vi "rotina_injecao_1.0.vi"() -> ()   [LabVIEW 2011]
panel:
  out "Cicles":i32
  in  "return valve (min)":dbl=1.1 caption="Time Target (s)"
  in  "#  Clicles":i32=3
  in  "stop air valve (s)":dbl=4.0 caption="Time Target (s)"
  in  "Time to get ready":dbl=0.5 caption="Time Target (s)"
  in  "Chromatogram Time (min)":dbl=2.0 caption="Time Target (s)"
  in  "Boolean":bool=TRUE
  out "TCD":dbl(graph)
  out "Time has Elapsed":bool
  out "Elapsed Time (min)":dbl caption="Elapsed Time (s)"
  out "Counter":i32
  out "FID":cluster{"value":dbl}(graph)
  out "date string":string
  out "time string":string
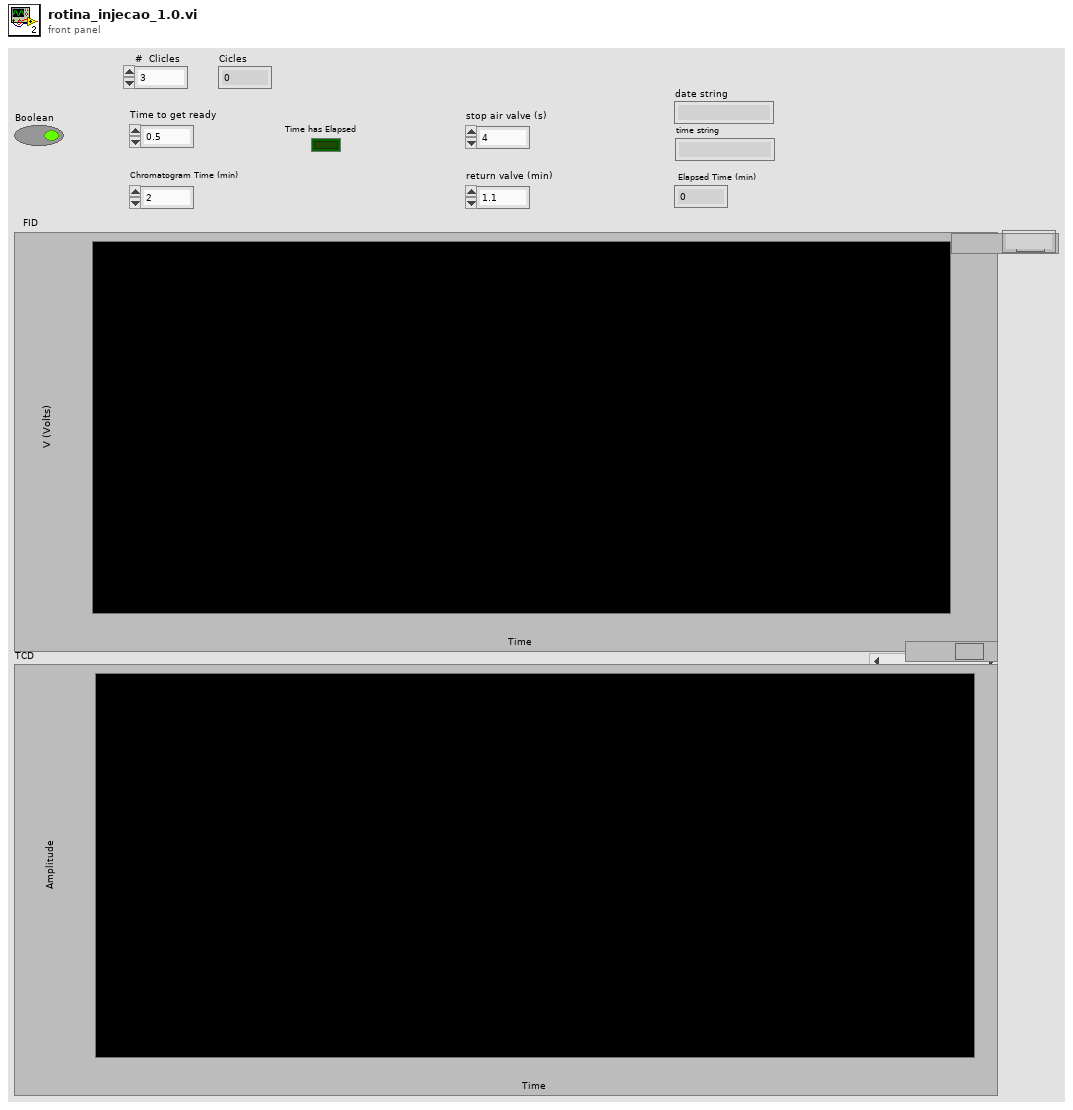
[diagram p1: front panel]
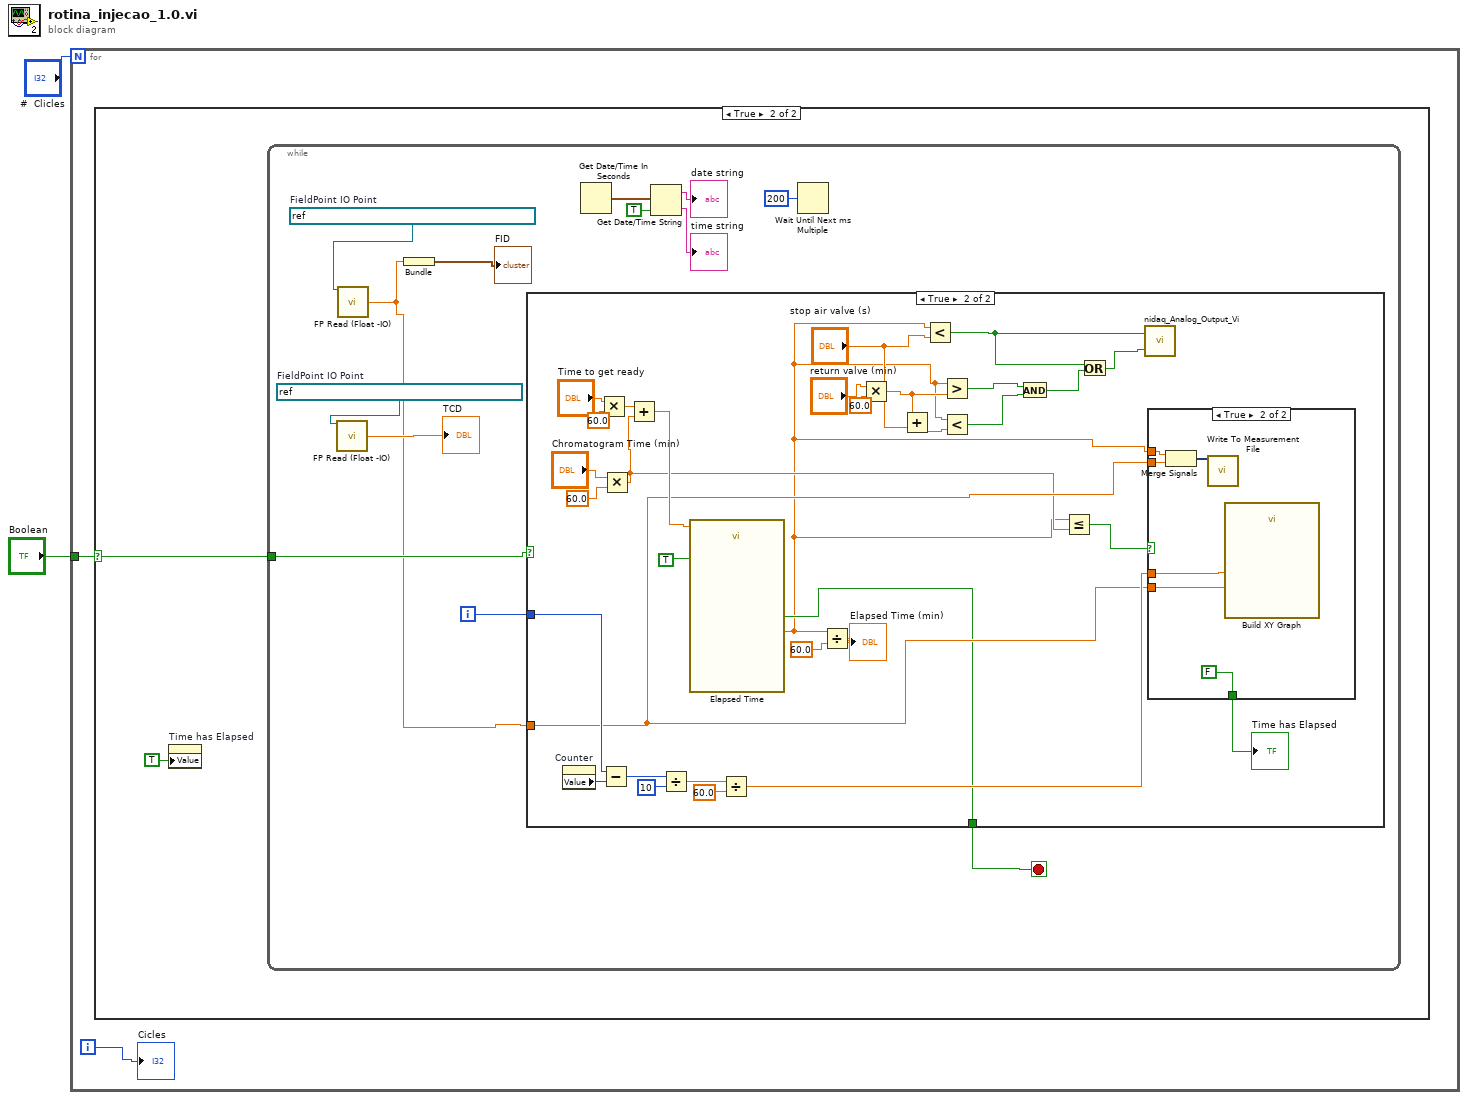
[diagram p0: block diagram]
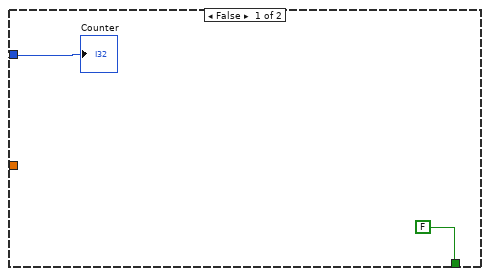
[diagram p3: hidden frame]
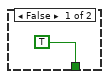
[diagram p4: hidden frame]
diagram:
  n1 = for {
    N: "#  Clicles" -> [_]
    tunnel: "Boolean" -> [w4]
    i -> [w3]
    n2 = case shown="True" w4 {
      selector: w4 -> [_ w5]
      frame False {
      }
      frame True {
        n3 = property on="Time has Elapsed" class="Bool (strict)"("Value"=TRUE ("Time has Elapsed")) -> ()  [unwired: 2 in, 2 out]
        n4 = while {
          tunnel: w5 -> [w13]
          i -> [w15]
          stop <- w7 stop-if-true
          w18 = refnum<k21> "FieldPoint\\cfp2220\\cFP-AI-110 @4\\Channel 2"  # FieldPoint IO Point
          w19 = refnum<k21> "FieldPoint\\cfp2220\\cFP-AI-110 @4\\Channel 0"  # FieldPoint IO Point
          n5 = call <vilib>:"FP Read (Float -IO).vi"("FieldPoint IO Point In"=w18) -> ("value"=→"TCD":dbl)  [unwired: 11 in, 3 out]
          n6 = call <vilib>:"FP Read (Float -IO).vi"("FieldPoint IO Point In"=w19) -> ("value"=w12:dbl)  [unwired: 11 in, 3 out]
          n7 = Bundle("value"=w12) -> (→"FID":cluster{"value":dbl})  [unwired: 1 out]
          n8 = case shown="True" w13 {
            tunnel: w12 -> [_ w38]
            tunnel: w15 -> [w21 w49]
            tunnel: [FALSE w37] -> w7
            frame False {
              "Counter" <- w21
            }
            frame True {
              n9 = property on="Counter" class="DigNum (strict)"() -> ("Value"=w48:i32)  [unwired: 2 in, 2 out]
              n10 = Multiply(x="Time to get ready", y=60.0) -> (x*y=w42:dbl)
              n11 = Subtract(x=w49, y=w48) -> (x-y=w50:i32)
              n12 = Multiply(x="Chromatogram Time (min)", y=60.0) -> (x*y=w23:dbl)
              n13 = Add(x=w42, y=w23) -> (x+y=w41:dbl)
              n14 = Divide(x=w50, y=10) -> (x/y=w52:dbl)
              n15 = call "Elapsed Time"("Time Target (s)"=w41, "Auto Reset"=TRUE) -> ("Elapsed Time (s)"=w22:dbl, "Time has Elapsed"=w37:bool)  [unwired: 10 in, 6 out]
              n16 = Divide(x=w52, y=60.0) -> (x/y=w39:dbl)
              n17 = Divide(x=w22, y=60.0) -> (x/y=→"Elapsed Time (min)":dbl)
              n18 = Multiply(x="return valve (min)", y=60.0) -> (x*y=w27:dbl)
              n19 = Add(x=w27, y="stop air valve (s)") -> (x+y=w28:dbl)
              n20 = Less?(x=w22, y="stop air valve (s)") -> (x < y?=w25:bool)
              n21 = Greater?(x=w22, y=w27) -> (0:w33:bool)
              n22 = Less?(x=w22, y=w28) -> (x < y?=w32:bool)
              n23 = And(x=w33, y=w32) -> (x .and. y?=w26:bool)
              n24 = Less Or Equal?(x=w22, y=w23) -> (x <= y?=w36:bool)
              n25 = Or(x=w25, y=w26) -> (x .or. y?=w24:bool)
              n26 = call "nidaq_Analog_Output_Vi.vi"("start Solenoide Valve"=w24, "start chromat"=w25) -> ()  [unwired: 1 in]
              n27 = case shown="True" w36 {
                tunnel: w22 -> [_ w59]
                tunnel: w38 -> [_ w58]
                tunnel: [TRUE FALSE] -> w40
                tunnel: w39 -> [_ w56]
                tunnel: w38 -> [_ w55]
                frame False {
                }
                frame True {
                  n28 = Merge Signals(w59, w58) -> (w60:dynamicdata)
                  n29 = call "Write To Measurement File"("Signals"=w60) -> ()  [unwired: 16 in, 3 out]
                  n30 = call "Build XY Graph"("Y Input"=w55, "X Input"=w56) -> ()  [unwired: 3 in, 7 out]
                }
              }
              "Time has Elapsed" <- w40
            }
          }
          n31 = Get Date/Time In Seconds() -> (seconds since 1Jan1904=w9:timestamp)
          n32 = Get Date/Time String(seconds (now)=w9, want seconds? (F)=TRUE) -> (date string=→"date string":string, time string=→"time string":string)  [unwired: 1 in]
          n33 = Wait Until Next ms Multiple(millisecond multiple=u32 200) -> ()  [unwired: 1 out]
        }
      }
    }
    "Cicles" <- w3
  }
